vi "ColorOrForce.vi"(6 "Port":string, 9 "note (input a number)":string, 10 "sensor":u16, 11 "String in":string) -> (3 "String out":string)   [LabVIEW 2022 SP3]
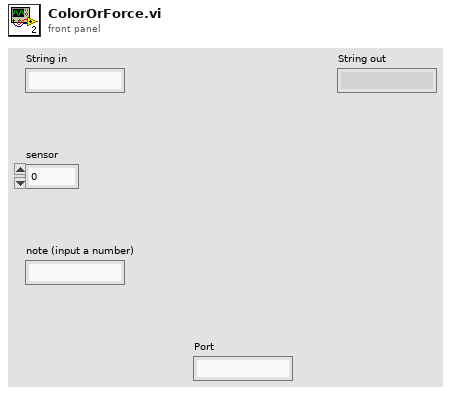
[diagram p1: front panel]
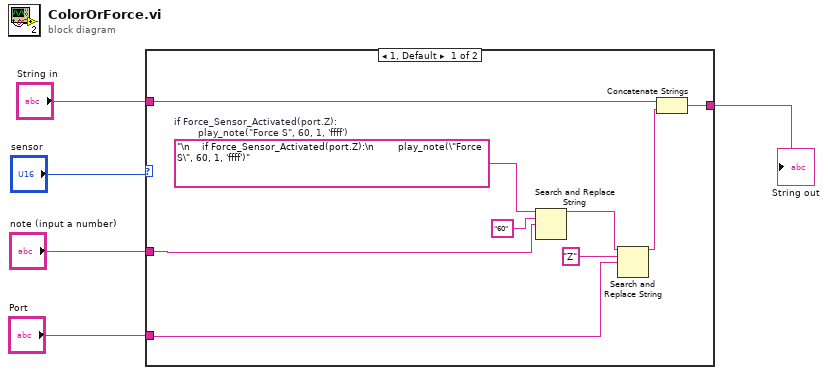
[diagram p0: block diagram]
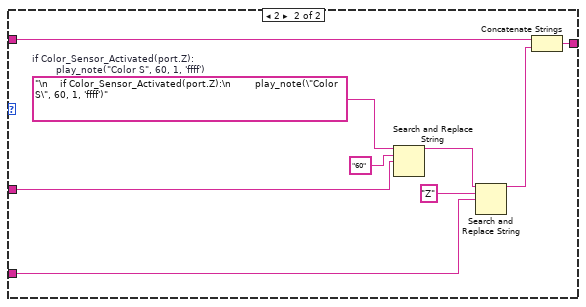
[diagram p2: hidden frame]
diagram:
  n1 = case shown="1, Default" "sensor" {
    tunnel: "String in" -> [w7 w23]
    tunnel: "note (input a number)" -> [w8 w20]
    tunnel: "Port" -> [w9 w19]
    tunnel: [w6 w15] -> w5
    frame 1, Default {
      w14 = "\n    if Force_Sensor_Activated(port.Z):\n        play_note(\"Force S\", 60, 1, 'ffff')"  # if Force_Sensor_Activated(port.Z):         play_note("Force S", 60, 1, 'ffff')
      n2 = Search and Replace String(input string=w14, search string="60", replace string=w8) -> (result string=w13:string)  [unwired: 5 in, 3 out]
      n3 = Search and Replace String(input string=w13, search string="Z", replace string=w9) -> (result string=w10:string)  [unwired: 5 in, 3 out]
      n4 = Concatenate Strings(w7, w10) -> (w6:string)
    }
    frame 2 {
      w22 = "\n    if Color_Sensor_Activated(port.Z):\n        play_note(\"Color S\", 60, 1, 'ffff')"  # if Color_Sensor_Activated(port.Z):         play_note("Color S", 60, 1, 'ffff')
      n5 = Search and Replace String(input string=w22, search string="60", replace string=w20) -> (result string=w21:string)  [unwired: 5 in, 3 out]
      n6 = Search and Replace String(input string=w21, search string="Z", replace string=w19) -> (result string=w16:string)  [unwired: 5 in, 3 out]
      n7 = Concatenate Strings(w23, w16) -> (w15:string)
    }
  }
  "String out" <- w5
